vi "Write Numeric.vi"(8 "error in (no error)":errorcluster, 10 "Numeric":dbl, 11 "ClassOutsideProject in":refnum<class "ClassOutsideProject.lvclass">) -> (0 "error out":errorcluster, 3 "ClassOutsideProject out":refnum<class "ClassOutsideProject.lvclass">)   [LabVIEW 2023, in "ClassOutsideProject.lvclass"]
uses:
  ClassOutsideProject.lvclass
  ClassOutsideProject.lvclass/ClassOutsideProject.ctl
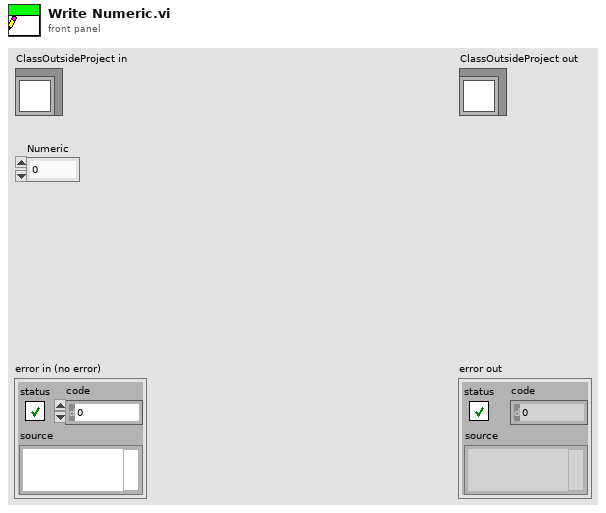
[diagram p1: front panel]
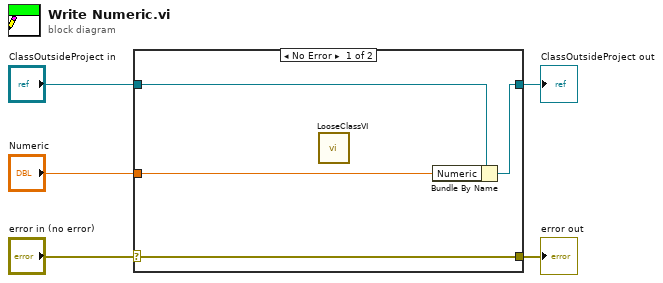
[diagram p0: block diagram]
diagram:
  n1 = case shown="No Error" "error in (no error)" {
    selector: "error in (no error)" -> [w9 w10]
    tunnel: [w9 w10] -> w4
    tunnel: [w7 w11] -> w2
    tunnel: "ClassOutsideProject in" -> [w8 w11]
    tunnel: "Numeric" -> [w6 _]
    frame No Error {
      n2 = call "LooseClassVI.vi"() -> ()  [unwired: 12 in]
      n3 = Bundle By Name(cluster=w8, "Numeric"=w6) -> (w7:refnum<class "ClassOutsideProject.lvclass">)
    }
    frame Error {
    }
  }
  "error out" <- w4
  "ClassOutsideProject out" <- w2
